vi "CRYAuto Create Recalled Waves.vi"(8 "all or last":i32, 9 "Curve Names in":string[](array[string]), 10 "Curves Selected?":bool[](array[boolean]), 11 "Wave array":T1[](array[typedef]) {"Y dB ref" format="%.1f"; "Y axis" items=["Log", "Lin"]; "Y data" items=["dB", "Lin"]; "X data" items=["dB", "Lin"]}) -> (3 "Wave Out":T1[](array[typedef]) {"Y dB ref" format="%.1f"; "Y axis" items=["Log", "Lin"]; "Y data" items=["dB", "Lin"]; "X data" items=["dB", "Lin"]})   [LabVIEW 2013]
uses:
  Typedef Control/CRYWaveform Cluster.ctl
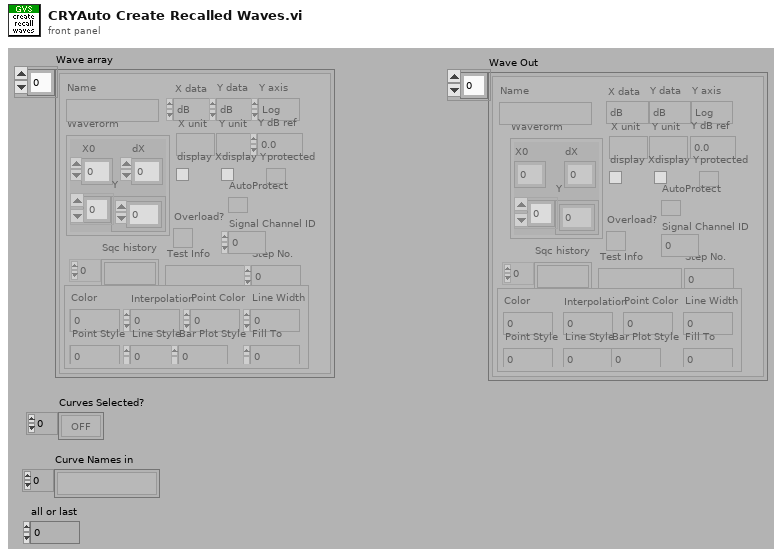
[diagram p1: front panel]
types:
  T1 = typedef "CRYWaveform Cluster.ctl" = cluster{"Waveform":cluster{"X0":dbl, "dX":dbl, "Y":sgl[]}, "X data":u16, "Y data":u16, "Y axis":u16, "X unit":string, "Y unit":string, "Y dB ref":dbl, "display Y":bool, "display X":bool, "Overload?":bool, "Test Info":string, "Step No.":i32, "Name":string, "protected":bool, "Sqc history":string[], "Signal Channel ID":i32, "Plot Settings":cluster{"Color":u32, "Interpolation":u8, "Point Style":u8, "Line Style":u8, "Point Color":u32, "Line Width":u8, "Bar Plot Style":u8, "Fill To":i16}, "AutoProtect":bool}
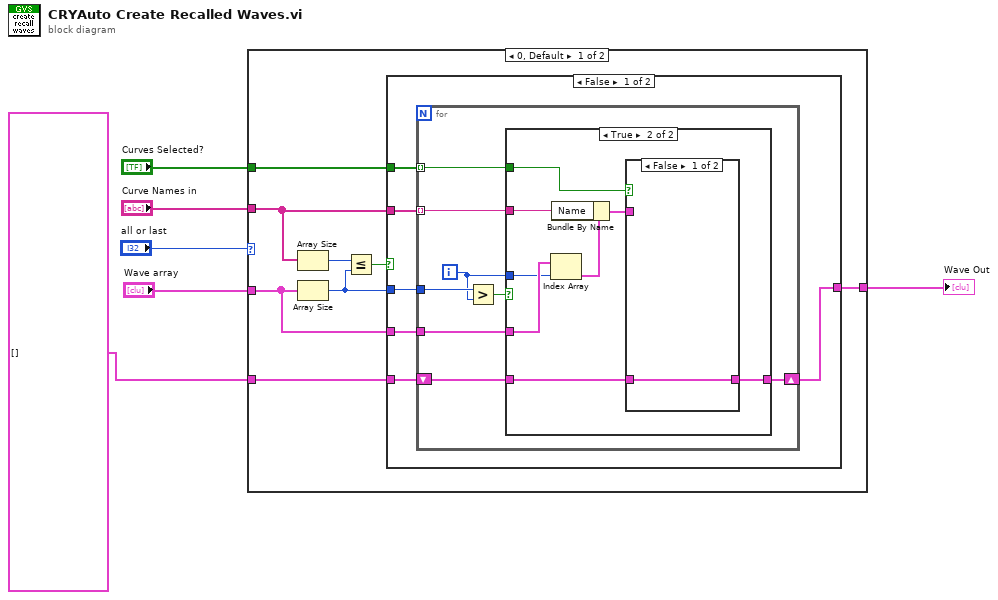
[diagram p0: block diagram]
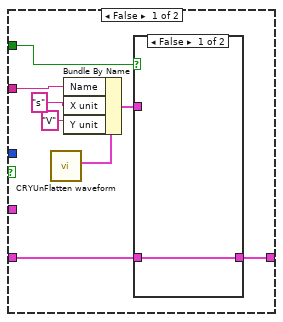
[diagram p2: hidden frame]
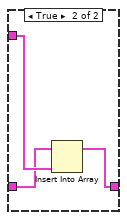
[diagram p3: hidden frame]
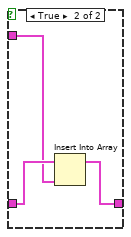
[diagram p4: hidden frame]
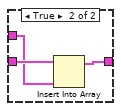
[diagram p6: hidden frame]
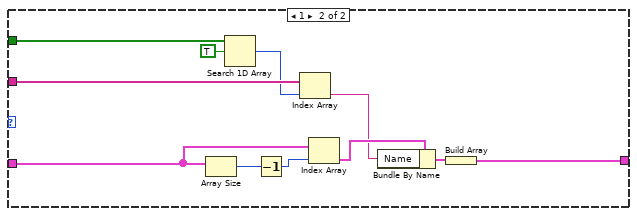
[diagram p7: hidden frame]
diagram:
  n1 = case shown="0, Default" "all or last" {
    tunnel: "Curve Names in" -> [w10 w73]
    tunnel: "Curves Selected?" -> [w12 w75]
    tunnel: T1[] [] ("appended array") -> [w11 _]
    tunnel: "Wave array" -> [w8 w66]
    tunnel: [w7 w65] -> w2
    frame 0, Default {
      n2 = Array Size(array=w10) -> (size(s)=w14:i32)
      n3 = Array Size(array=w8) -> (size(s)=w9:i32)
      n4 = Less Or Equal?(x=w14, y=w9) -> (x <= y?=w13:bool)
      n5 = case shown="False" w13 {
        tunnel: w12 -> [w20 w56]
        tunnel: w8 -> [w17 w55]
        tunnel: w11 -> [w16 w54]
        tunnel: w10 -> [w19 _]
        tunnel: [w15 w53] -> w7
        tunnel: w9 -> [w18 _]
        frame False {
          n6 = for {
            tunnel: w20 -> [w26] mode=indexing
            tunnel: w19 -> [w23] mode=indexing
            tunnel: w18 -> [w28]
            tunnel: w17 -> [w25]
            shift-right: [w21] -> w15
            shift-left: w16 -> [w22]
            i -> [w24]
            n7 = Greater?(x=w28, y=w24) -> (0:w27:bool)
            n8 = case shown="True" w27 {
              tunnel: w26 -> [w36 w48]
              tunnel: w25 -> [_ w47]
              tunnel: w24 -> [_ w46]
              tunnel: w23 -> [w35 w44]
              tunnel: w22 -> [w31 w42]
              tunnel: [w30 w41] -> w21
              frame False {
                n9 = call "CRYUnFlatten waveform.vi"() -> ("Waveform Cluster"=w29:T1)  [unwired: 9 in, 2 out]
                n10 = Bundle By Name(cluster=w29, "Name"=w35, "X unit"="s", "Y unit"="V" ("Z unit")) -> (w32:T1)
                n11 = case shown="False" w36 {
                  tunnel: w32 -> [_ w40]
                  tunnel: w31 -> [w37 w39]
                  tunnel: [w37 w38] -> w30
                  frame False {
                  }
                  frame True {
                    n12 = Insert Into Array(array=w39, new element=w40) -> (w38:T1[])  [unwired: 1 in]
                  }
                }
              }
              frame True {
                n13 = Index Array(array=w47, index=w46) -> (element=w45:T1)
                n14 = Bundle By Name(cluster=w45, "Name"=w44) -> (w43:T1)
                n15 = case shown="False" w48 {
                  tunnel: w43 -> [_ w51]
                  tunnel: w42 -> [w49 w52]
                  tunnel: [w49 w50] -> w41
                  frame False {
                  }
                  frame True {
                    n16 = Insert Into Array(array=w52, new element=w51) -> (w50:T1[])  [unwired: 1 in]
                  }
                }
              }
            }
          }
        }
        frame True {
          n17 = for {
            tunnel: w56 -> [w60] mode=indexing
            tunnel: w55 -> [w57] mode=indexing
            shift-right: [w58] -> w53
            shift-left: w54 -> [w59]
            n18 = case shown="False" w60 {
              tunnel: w57 -> [_ w63]
              tunnel: w59 -> [w61 w64]
              tunnel: [w61 w62] -> w58
              frame False {
              }
              frame True {
                n19 = Insert Into Array(array=w64, new element=w63) -> (w62:T1[])  [unwired: 1 in]
              }
            }
          }
        }
      }
    }
    frame 1 {
      n20 = Array Size(array=w66) -> (size(s)=w71:i32)
      n21 = Search 1D Array(1D array=w75, element=TRUE) -> (index of element=w72:i32)  [unwired: 1 in]
      n22 = Decrement(x=w71) -> (x-1=w70:i32)
      n23 = Index Array(array=w73, index=w72) -> (element=w68:string)
      n24 = Index Array(array=w66, index=w70) -> (element=w69:T1)
      n25 = Bundle By Name(cluster=w69, "Name"=w68) -> (w67:T1)
      n26 = Build Array(w67) -> (w65:T1[])
    }
  }
  "Wave Out" <- w2
